vi "LaunchMain.vi"(0 "ActionsOnEvents in":refnum<class "ActionsOnEvents.lvclass">, 1 "ActionsClass":string, 2 "Events":T1, 3 "IniFile":path=path "a3s/ini", 5 "error in (no error)":errorcluster) -> (14 "ActionsOnEvents out":refnum<class "ActionsOnEvents.lvclass">, 19 "error out":errorcluster)   [LabVIEW 2017, in "ActionsOnEvents.lvclass"]
uses:
  ActionsOnEvents.lvclass
  SystemEventData/SystemEventsType.ctl
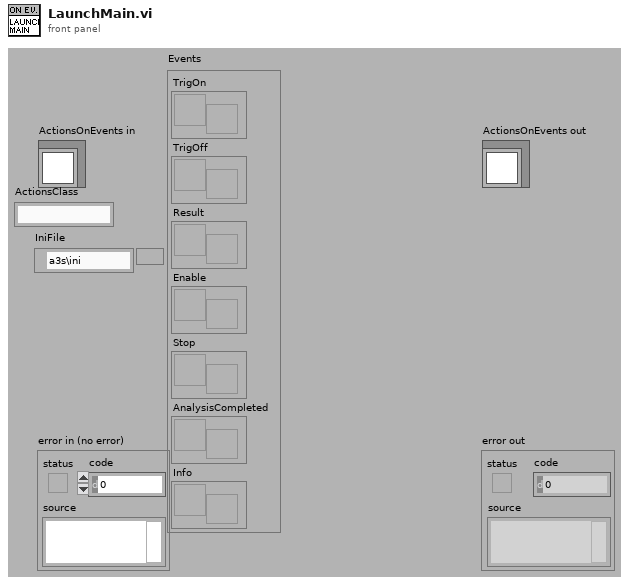
[diagram p1: front panel]
types:
  T1 = typedef "SystemEventsType.ctl" = cluster{"TrigOn":refnum<user-event>, "TrigOff":refnum<user-event>, "Result":refnum<user-event>, "Enable":refnum<user-event>, "Stop":refnum<user-event>, "AnalysisCompleted":refnum<user-event>, "Info":refnum<user-event>}
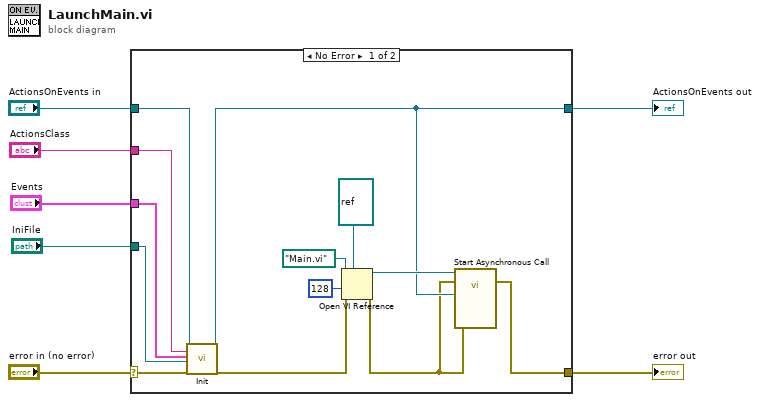
[diagram p0: block diagram]
diagram:
  n1 = case shown="No Error" "error in (no error)" {
    selector: "error in (no error)" -> [w20 w22]
    tunnel: [w8 w22] -> w6
    tunnel: [w10 w21] -> w4
    tunnel: "ActionsOnEvents in" -> [w18 w21]
    tunnel: "ActionsClass" -> [w17 _]
    tunnel: "Events" -> [w16 _]
    tunnel: "IniFile" -> [w13 _]
    frame No Error {
      n2 = call "Init.vi"("ActionsOnEvents in"=w18, "ActionsClass"=w17, "Events"=w16, "IniFile"=w13, "error in (no error)"=w20) -> ("ActionsOnEvents out"=w10:refnum<class "ActionsOnEvents.lvclass">, "error out"=w19:errorcluster)  [unwired: 13 in]
      n3 = Open VI Reference(type specifier VI Refnum (for type only)=refnum<vi> refnum, vi path=path "Main.vi", options=128, error in (no error)=w19) -> (vi reference=w11:refnum<vi>, error out=w9:errorcluster)  [unwired: 1 in, 1 out]
      n4 = call-by-ref "Start Asynchronous Call"(reference=w11, error in=w9, "ActionsOnEvents in"=w10, 5:"error in (no error)"=w9) -> (error out=w8:errorcluster)  [unwired: 16 in, 3 out]
    }
    frame Error {
    }
  }
  "error out" <- w6
  "ActionsOnEvents out" <- w4
